vi "SetSpeed.vi"(8 "error in (no error)":errorcluster, 10 "Input: Speed in microns/sec":i32, 11 "Serial Controller in":refnum<class "Serial Controller.lvclass">) -> (0 "error out":errorcluster, 1 "Read":bool, 2 "Output: Speed in microns/sec":u32, 3 "Serial Controller out":refnum<class "Serial Controller.lvclass">)   [LabVIEW 2014, in "Serial Controller.lvclass"]
uses:
  Serial Controller.lvclass
  Serial Controller.lvclass/Serial Controller.ctl
panel:
  out "Serial Read":string
  out "Word to MP-285":string
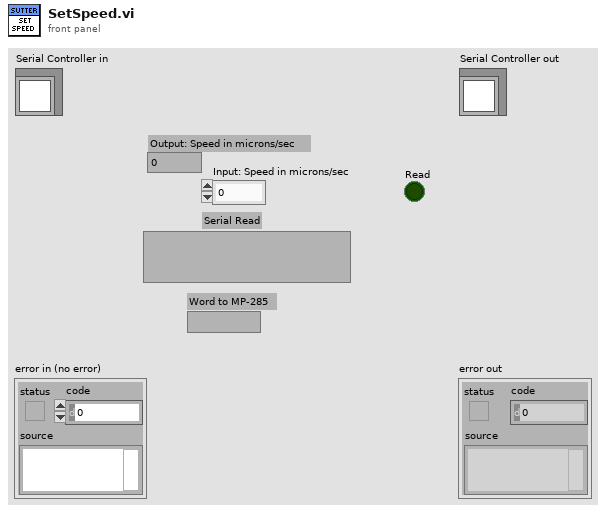
[diagram p1: front panel]
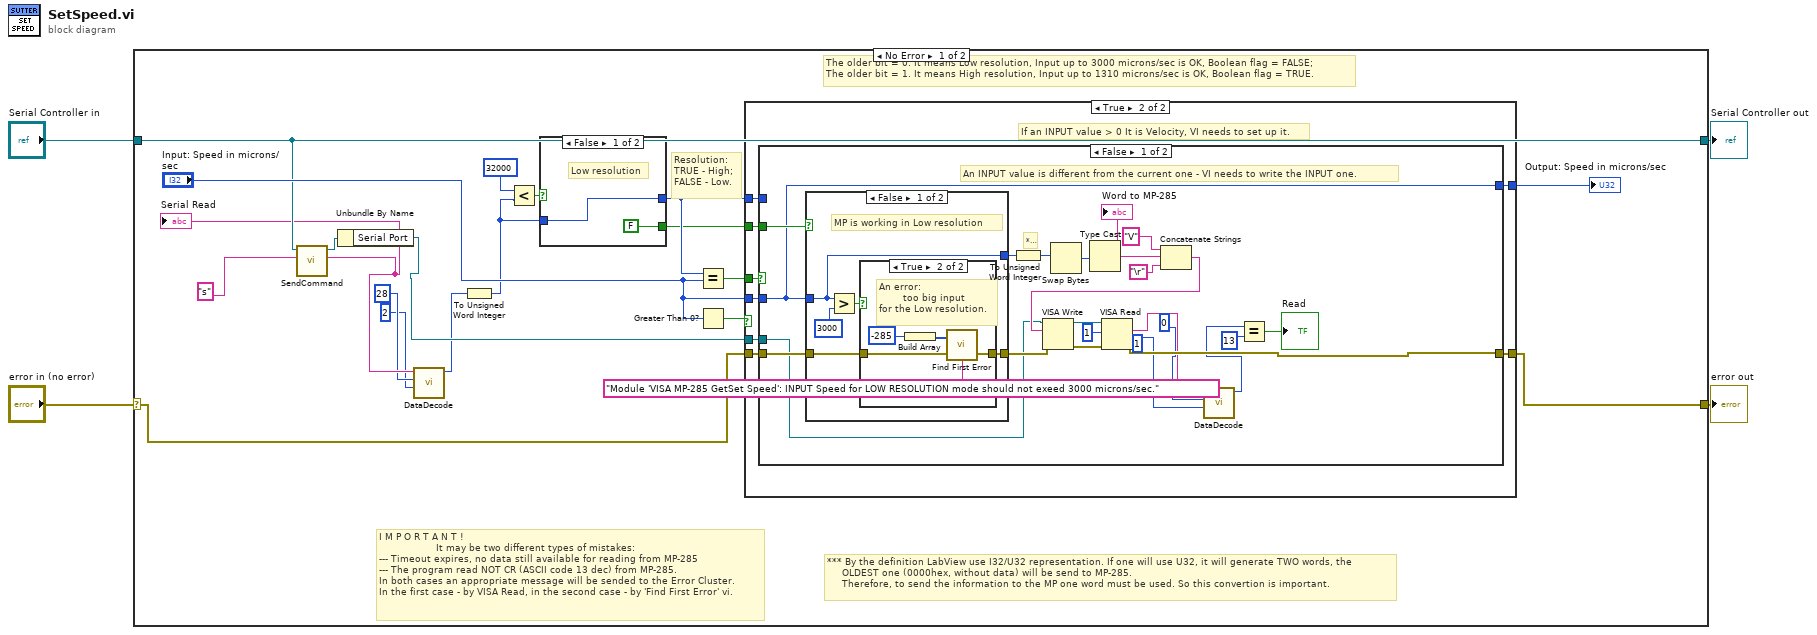
[diagram p0: block diagram]
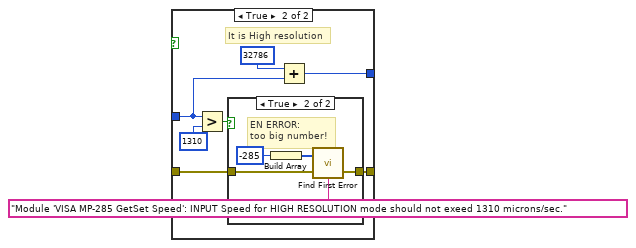
[diagram p4: hidden frame]
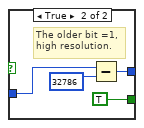
[diagram p7: hidden frame]
diagram:
  n1 = case shown="No Error" "error in (no error)" {
    selector: "error in (no error)" -> [w10 w89]
    tunnel: [w9 w89] -> w3
    tunnel: [w13 w88] -> w1
    tunnel: "Serial Controller in" -> [w13 w88]
    frame No Error {
      # "*** By the definition LabView use I32/U32 representation. If one will use U32, it will generate TWO words, the \n     OLDEST one (0000hex, without data) will be send to MP-285. \n     Therefore, to send the information to the MP one word must be used. So this convertion is important."
      # "The older bit = 0. It means Low resolution, Input up to 3000 microns/sec is OK, Boolean flag = FALSE;\nThe older bit = 1. It means High resolution, Input up to 1310 microns/sec is OK, Boolean flag = TRUE."
      # "Resolution:\nTRUE - High;\nFALSE - Low."
      # "I M P O R T A N T !\n                   It may be two different types of mistakes: \n--- Timeout expires, no data still available for reading from MP-285\n--- The program read NOT CR (ASCII code 13 dec) from MP-285.\nIn both cases an appropriate message will be sended to the Error Cluster.\nIn the first case - by VISA Read, in the second case - by 'Find First Error' vi."
      n2 = call-dynamic "SendCommand.vi"("command"="s", "Serial Controller in"=w13) -> ("Returned"=w8:string, "Serial Controller out"=w12:refnum<class "Serial Controller.lvclass">)  [unwired: 7 in, 1 out]
      "Serial Read" <- w8
      n3 = Unbundle By Name(w12) -> ("Serial Port"=w11:refnum<visa-resource-name>)
      n4 = call "DataDecode.vi"("Input: lenght"=2 ("length"), "Input: offset"=28 ("offset (0)"), "Input: Data string"=w8) -> ("Output: Decoded Data"=w5:i32)  [unwired: 4 in]
      n5 = To Unsigned Word Integer(number=w5) -> (unsigned 16bit integer=w17:u16)
      n6 = Less?(x=32000, y=w17) -> (x < y?=w15:bool)
      n7 = case shown="False" w15 {
        tunnel: [w83 w87] -> w22
        tunnel: w17 -> [w83 w85]
        tunnel: [FALSE TRUE] -> w19
        frame False {
          # "Low resolution"
        }
        frame True {
          # "The older bit =1, \nhigh resolution."
          n8 = Subtract(x=w85, y=32786) -> (x-y=w87:i32)
        }
      }
      n9 = Equal?(x=w22, y="Input: Speed in microns/sec") -> (x = y?=w18:bool)
      n10 = Greater Than 0?(x="Input: Speed in microns/sec") -> (x > 0?=w20:bool)
      n11 = case shown="True" w20 {
        tunnel: w11 -> [_ w33]
        tunnel: w10 -> [w25 w32]
        tunnel: w18 -> [_ w31]
        tunnel: [w25 w30] -> w9
        tunnel: w19 -> [_ w29]
        tunnel: "Input: Speed in microns/sec" -> [_ w28]
        tunnel: w22 -> [w24 w27]
        tunnel: [w24 w26] -> w23
        frame False {
          # "If an INPUT value <=0 there is nothing to write, just output the current Velocity."
        }
        frame True {
          # "If an INPUT value > 0 It is Velocity, VI needs to set up it."
          n12 = case shown="False" w31 {
            tunnel: w32 -> [w54 w81]
            tunnel: w33 -> [w47 _]
            tunnel: [w38 w81] -> w30
            tunnel: w29 -> [w55 _]
            tunnel: w28 -> [w40 _]
            tunnel: w27 -> [_ w80]
            tunnel: [w40 w80] -> w26
            frame False {
              # "***"
              # "An INPUT value is different from the current one - VI needs to write the INPUT one."
              n13 = case shown="False" w55 {
                tunnel: w40 -> [w60 w70]
                tunnel: w54 -> [w57 w71]
                tunnel: [w60 w68] -> w42
                tunnel: [w56 w67] -> w48
                frame False {
                  # "MP is working in Low resolution"
                  n14 = Greater?(x=w60, y=3000) -> (0:w58:bool)
                  n15 = case shown="True" w58 {
                    tunnel: w57 -> [w61 w66]
                    tunnel: [w61 w65] -> w56
                    frame False {
                      # "An INPUT is\nin range."
                    }
                    frame True {
                      # "An error:\n        too big input\nfor the Low resolution."
                      n16 = Build Array(-285) -> (w63:i32[])
                      n17 = call <vilib>:"Find First Error.vi"("error in (no error)"=w66, "source messages"="Module 'VISA MP-285 GetSet Speed': INPUT Speed for LOW RESOLUTION mode should not exeed 3000 microns/sec.", "error codes"=w63) -> ("error out"=w65:errorcluster)  [unwired: 2 out]
                    }
                  }
                }
                frame True {
                  # "It is High resolution"
                  n18 = Greater?(x=w70, y=1310) -> (0:w72:bool)
                  n19 = case shown="True" w72 {
                    tunnel: w71 -> [w74 w78]
                    tunnel: [w74 w79] -> w67
                    frame False {
                      # "Input correct, \nWe can write."
                    }
                    frame True {
                      # "EN ERROR:\ntoo big number!"
                      n20 = Build Array(-285) -> (w76:i32[])
                      n21 = call <vilib>:"Find First Error.vi"("error in (no error)"=w78, "source messages"="Module 'VISA MP-285 GetSet Speed': INPUT Speed for HIGH RESOLUTION mode should not exeed 1310 microns/sec.", "error codes"=w76) -> ("error out"=w79:errorcluster)  [unwired: 2 out]
                    }
                  }
                  n22 = Add(x=32786, y=w70) -> (x+y=w68:i32)
                }
              }
              n23 = To Unsigned Word Integer(number=w42) -> (unsigned 16bit integer=w41:u16)
              n24 = Swap Bytes(anything=w41) -> (byte swapped=w44:u16)
              n25 = Type Cast(x=w44) -> (*(type *) &x=w43:string)  [unwired: 1 out]
              "Word to MP-285" <- w43
              n26 = Concatenate Strings("V", w43, "\r") -> (w52:string)
              n27 = VISA Write(VISA resource name=w47, write buffer=w52, error in (no error)=w48) -> (VISA resource name out=w51:refnum<visa-resource-name>, error out=w50:errorcluster)  [unwired: 1 out]
              n28 = VISA Read(VISA resource name=w51, byte count=1, error in (no error)=w50) -> (read buffer=w37:string, error out=w38:errorcluster)  [unwired: 2 out]
              n29 = call "DataDecode.vi"("Input: lenght"=1, "Input: offset"=0, "Input: Data string"=w37) -> ("Output: Decoded Data"=w34:i32)  [unwired: 4 in]
              n30 = Equal?(x=w34, y=13) -> (x = y?=→"Read":bool)
            }
            frame True {
              # "An INPUT value is the same, as current one --> Nothing to do!"
            }
          }
        }
      }
      "Output: Speed in microns/sec" <- w23
    }
    frame Error {
    }
  }
  "error out" <- w3
  "Serial Controller out" <- w1
